vi "zahvat.vi"   [LabVIEW 2017]
uses:
  <vilib>/myRIO/Common/Instrument Driver Framework/myRIO v1.0/UART/vis/myRIO v1.0 Close UART.vi
  <vilib>/myRIO/Common/Instrument Driver Framework/Utilities/vis/FPGA Ref Manager.vi
  <vilib>/myRIO/Common/Instrument Driver Framework/myRIO v1.0/myRIO v1.0 Reset FPGA.vi
  <vilib>/myRIO/Common/Instrument Driver Framework/myRIO v1.0/IRQ/vis/myRIO v1.0 IRQ Info FGV.vi
  <vilib>/myRIO/Common/Instrument Driver Framework/myRIO v1.0/IRQ/vis/myRIO v1.0 Timer IRQ Info FGV.vi
  <vilib>/myRIO/Common/Instrument Driver Framework/myRIO v1.0/IRQ/vis/myRIO v1.0 ISR Agent.vi
  <vilib>/myRIO/Instrument Drivers/Utilities/Utilities.lvlib
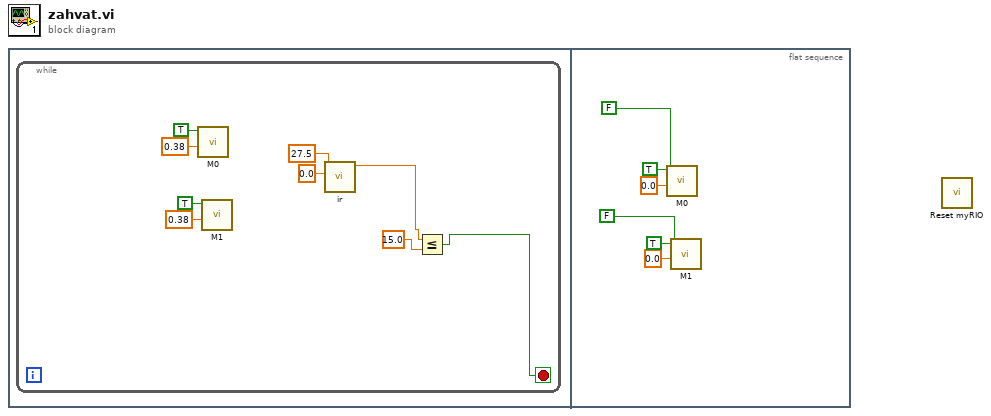
[diagram p0: block diagram]
diagram:
  n1 = flat-sequence {
    frame #0 {
      n2 = while {
        stop <- w4 stop-if-true
        n3 = call "M0.vi"("Duty Cycle"=0.38, "вперед"=TRUE) -> ()  [unwired: 9 in, 1 out]
        n4 = call "M1.vi"("Duty Cycle"=0.38, "вперед"=TRUE) -> ()  [unwired: 9 in, 1 out]
        n5 = call "ir.vi"("Koffset [cm]"=0.0, "Kscale [cm-V]"=27.5) -> ("см"=w3:dbl)  [unwired: 8 in, 1 out]
        n6 = Less Or Equal?(x=w3, y=15.0) -> (x <= y?=w4:bool)
      }
    }
    frame #1 {
      n7 = call "M0.vi"("Duty Cycle"=0.0, "назад"=FALSE, "вперед"=TRUE) -> ()  [unwired: 8 in, 1 out]
      n8 = call "M1.vi"("Duty Cycle"=0.0, "назад"=TRUE ("вперед"), "вперед"=FALSE ("назад")) -> ()  [unwired: 8 in, 1 out]
    }
  }
  n9 = call <vilib>:"Reset myRIO.vi"() -> ()  [unwired: 11 in, 1 out]
